vi "ROI group-Event handler-ROI group mouse move.vi"(9 "Coords":T2, 11 "[Groups]":T1) -> (0 "error out":errorcluster)   [LabVIEW 2017]
uses:
  <vilib>/Utility/miscctls.llb/LVPoint32TypeDef.ctl
  Typedefs/Groups array referecne.ctl
  Global variables/gl_Functional Imaging-Global variables.vi
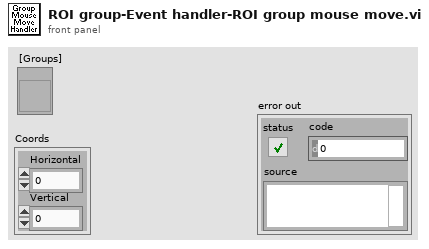
[diagram p1: front panel]
types:
  T1 = typedef "Groups array referecne.ctl" = refnum<vi>
  T2 = typedef "LVPoint32TypeDef.ctl" = cluster{"Horizontal":i32, "Vertical":i32}
  T3 = typedef "Functional Imging UI Refs.ctl" = cluster{"Menu ref":refnum<k9>, "Image control":refnum<vi>, "VI ref":refnum<vi>, "XGrapher":refnum<vi>, "Smoothing":refnum<vi>, "POI Averaging":refnum<vi>, "Normalize":refnum<vi>, "POI data points in each trial":refnum<vi>, "Channel":refnum<vi>, "Experiment data folder path":refnum<vi>, "[ROI vis]":refnum<vi>, "[Groups] visbl":T1, "Group Name":refnum<vi>, "POI index":refnum<vi>, "Trial No.":refnum<vi>, "Intensity Zoom":refnum<vi>, "Trial Cursor Enabled":refnum<vi>, "Number of Trials (ind 1)":refnum<vi>, "Number of Trials (ind 2)":refnum<vi>, "MiniScans Available":refnum<vi>, "POI Available":refnum<vi>, "Defer graph updates":refnum<vi>, "Waveform selector":refnum<vi>, "#of selected POI":refnum<vi>, "#of selected MiniScans":refnum<vi>, "#of selected groups":refnum<vi>, "Max Z-Projection":refnum<vi>, "Z-Plane Selector":refnum<vi>, "Index of miniscan point to visualise":refnum<vi>, "ROI vis. mode":refnum<vi>, "Total # of points":refnum<vi>, "Index of group clicked on":refnum<vi>, "Pane 1":refnum<vi>, "Pane 2":refnum<vi>, "Pane 3":refnum<vi>, "Pane 4":refnum<vi>, "Pane 5":refnum<vi>, "Pane 6":refnum<vi>, "Deselect all ROI":refnum<vi>, "Deselect all groups":refnum<vi>}
  T4 = typedef "Group sel cluster.ctl" = cluster{"Group number":string, "Group Name":string, "Visibility":bool, "Highlight":bool}
  T5 = typedef "ROI group info cluster.ctl" = cluster{"Group name":string, "# ROI in group":i32, "ROI numbers in group":i32[], "Group region specifier cluster":T6}
  T6 = typedef "ROI Descriptor" = cluster{"Global Rectangle":i32[], "Contours":cluster{"ID":enum32{"External", "Internal"}, "Type":u32, "Coordinates":i32[]}[]}
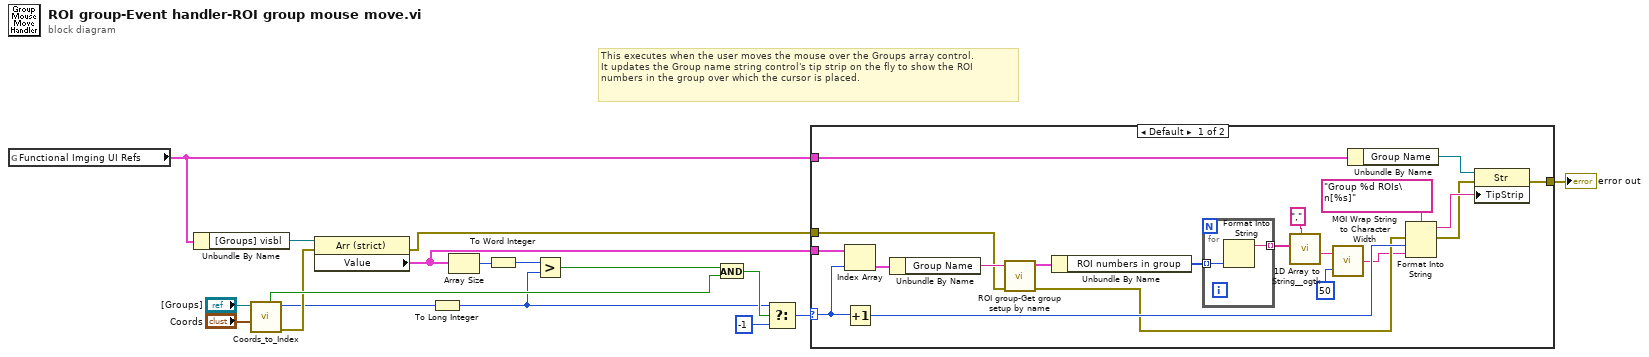
[diagram p0: block diagram]
diagram:
  # "This executes when the user moves the mouse over the Groups array control.\nIt updates the Group name string control's tip strip on the fly to show the ROI numbers in the group over which the cursor is placed."
  n1 = global read "gl_Functional Imaging-Global variables.vi" "Functional Imging UI Refs"() -> (w5:T3)
  n2 = Unbundle By Name(w5) -> ("[Groups] visbl"=w14:T1)
  n3 = call "Coords_to_Index.vi"("coords"="Coords", "Array ref"="[Groups]") -> ("error out"=w9:errorcluster, "row index"=w8:i16, "V In Range?"=w11:bool)  [unwired: 5 in, 2 out]
  n4 = property on="Property Node" class="Arr (strict)"(reference=w14, error in=w9) -> (error out=w2:errorcluster, "Value"=w4:T4[])  [unwired: 1 out]
  n5 = To Long Integer(number=w8) -> (32bit integer=w3:i32)
  n6 = Array Size(array=w4) -> (size(s)=w13:i32)
  n7 = To Word Integer(number=w13) -> (16bit integer=w7:i16)
  n8 = Greater?(x=w7, y=w3) -> (0:w12:bool)
  n9 = And(x=w12, y=w11) -> (x .and. y?=w10:bool)
  n10 = Select(t=w3, s=w10, f=-1) -> (s? t:f=w6:i32)
  n11 = case shown="Default" w6 {
    selector: w6 -> [w25 _]
    tunnel: w5 -> [w37 _]
    tunnel: w4 -> [w36 _]
    tunnel: w2 -> [w33 w40]
    tunnel: [w26 w40] -> w1
    frame Default {
      n12 = Index Array(array=w36, index=w25) -> (element=w35:T4)
      n13 = Increment(x=w25) -> (x+1=w23:i32)
      n14 = Unbundle By Name(w35) -> ("Group Name"=w34:string)
      n15 = call "ROI group-Get group setup by name.vi"("error in"=w33, "Name of ROI group to search for"=w34) -> ("error out (no error)"=w22:errorcluster, "POI group info cluster"=w32:T5)  [unwired: 7 in, 1 out]
      n16 = Unbundle By Name(w32) -> ("ROI numbers in group"=w31:i32[])
      n17 = for {
        tunnel: w31 -> [w39] mode=indexing
        tunnel: [w38] -> w30 mode=indexing
        n18 = Format Into String(w39) -> (resulting string=w38:string)  [unwired: 3 in, 1 out]
      }
      n19 = call <userlib>:"1D Array to String__ogtk.vi"("delimiter (Tab)"=",", "Array of Strings"=w30) -> ("delimited string"=w20:string)  [unwired: 9 in]
      n20 = call <userlib>:"MGI Wrap String to Character Width.vi"("Wrap length(Characters)"=50, "Unwrapped string"=w20) -> ("Wrapped String"=w19:string)
      n21 = Unbundle By Name(w37) -> ("Group Name"=w18:refnum<vi>)
      n22 = Format Into String(format string="Group %d ROIs\n[%s]" ("initial string"), error in=w22, w23, w19) -> (resulting string=w28:string, error out=w27:errorcluster)  [unwired: 1 in]
      n23 = property class="Str"(reference=w18, error in=w27, "TipStrip"=w28) -> (error out=w26:errorcluster)  [unwired: 1 out]
    }
    frame -1 {
    }
  }
  "error out" <- w1
